vi "Initialize.vi"(8 "error in (no error)":errorcluster, 11 "GW-PickUp-Cmd in":refnum<class "GW-PickUp-Cmd.lvclass">) -> (0 "error out":errorcluster, 3 "GW-PickUp-Cmd out":refnum<class "GW-PickUp-Cmd.lvclass">)   [LabVIEW 2013, in "GW-PickUp-Cmd.lvclass"]
uses:
  GW-PickUp-Cmd.lvclass
  States/GW-PickingUp-State/GW-PickingUp-State.lvclass
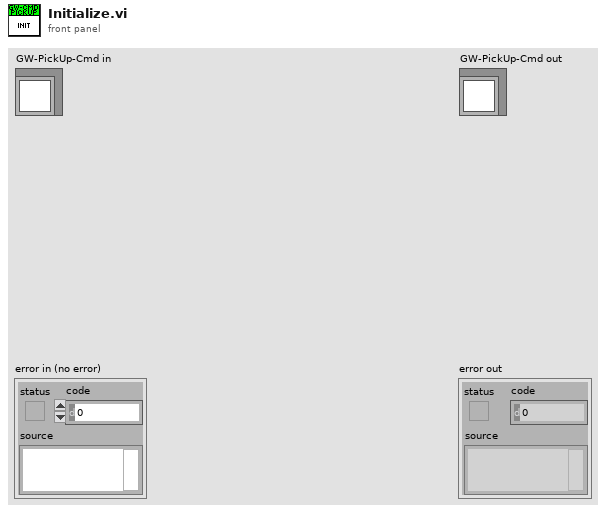
[diagram p1: front panel]
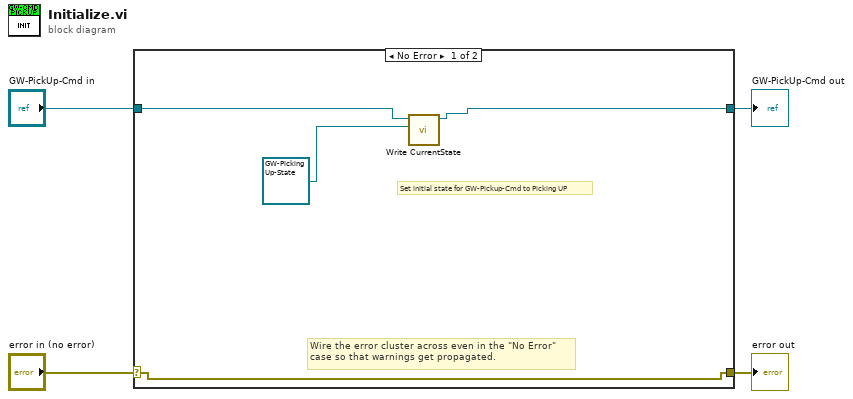
[diagram p0: block diagram]
diagram:
  n1 = case shown="No Error" "error in (no error)" {
    selector: "error in (no error)" -> [w6 w10]
    tunnel: [w6 w10] -> w3
    tunnel: [w7 w9] -> w1
    tunnel: "GW-PickUp-Cmd in" -> [w8 w9]
    frame No Error {
      # "Set initial state for GW-Pickup-Cmd to Picking UP"
      # "Wire the error cluster across even in the \"No Error\"\ncase so that warnings get propagated."
      n2 = call-dynamic "Write CurrentState.vi"("State.lvclass"=refnum<class "GW-PickingUp-State.lvclass"> refnum ("GW-PickingUp-State.lvclass"), "Command in"=w8) -> ("Command out"=w7:refnum<class "GW-PickUp-Cmd.lvclass">)  [unwired: 8 in, 1 out]
    }
    frame Error {
    }
  }
  "error out" <- w3
  "GW-PickUp-Cmd out" <- w1
